vi "WPI_JoystickFindJoystick.vi"(8 "error in (no error)":errorcluster, 9 "Joystick Info":T3, 11 "Match Criteria":T2(array[ring])) -> (0 "error out":errorcluster, 2 "Matching Joysticks":T1[](array[typedef]))   [LabVIEW 2017]
doc: "Search, and return the joystick indices that match the specified criteria.\nName includes is case agnostic, counts match of greater or equal to the critera, and Axis types matches if all criteria are present.\n\nThis software is licensed. Open the labview\\readme\\WPI Robotics Library Open Source License.txt file for more information."
uses:
  <vilib>/Rock Robotics/WPI/Joystick/WPI_Joystick Info.ctl
  <vilib>/Rock Robotics/WPI/Joystick/WPI_JoystickHID Types.ctl
  <vilib>/Rock Robotics/WPI/Joystick/WPI_JoystickXBox Types.ctl
  <vilib>/Rock Robotics/WPI/Joystick/WPI_JoystickAxis Types.ctl
  <vilib>/Rock Robotics/WPI/Joystick/WPI_JoystickDeviceEnum.ctl
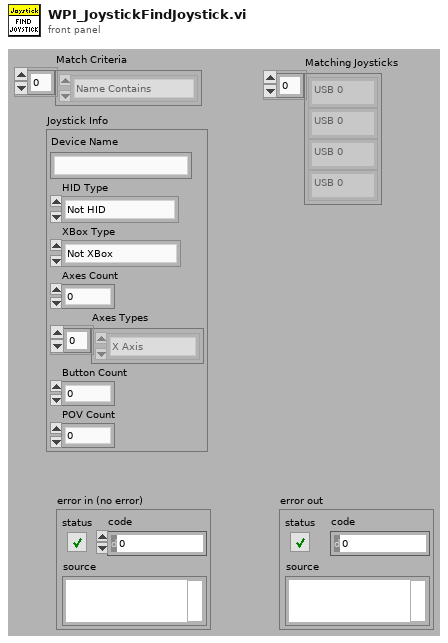
[diagram p1: front panel]
types:
  T1 = typedef "WPI_JoystickDeviceEnum.ctl" = enum16{"USB 0", "USB 1", "USB 2", "USB 3", "USB 4", "USB 5"}
  T2 = enum16{"Name Contains", "Name Equals", "HID Type", "XBox Type", "Axis Count", "Axis Type", "Button Count", "POV Count"}[]
  T3 = typedef "WPI_Joystick Info.ctl" = cluster{"Device Name":string, "HID Type":T4, "XBox Type":T5, "Axes Count":i32, "Axes Types":T6[], "Button Count":i32, "POV Count":i32}
  T4 = typedef "WPI_JoystickHID Types.ctl" = enum16{"Not HID", "HID Joystick", "HID Gamepad", "HID Driving Wheel", "HID Flightstick", "HID First Person"}
  T5 = typedef "WPI_JoystickXBox Types.ctl" = enum16{"Not XBox", "XBox Unknown", "XBox Gamepad", "XBox Wheel", "XBox Arcade Stick", "XBox Flight Stick", "XBox Dance Pad", "XBox Guitar", "XBox Drum Kit", "XBox Arcade Pad"}
  T6 = typedef "WPI_JoystickAxis Types.ctl" = enum16{"X Axis", "Y Axis", "Z Axis", "RxAxis", "RyAxis", "RzAxis", "Slider", "POV", "None", "L X Axis", "L Y Axis", "L Trigger", "R Trigger", "R X Axis", "R Y Axis"}
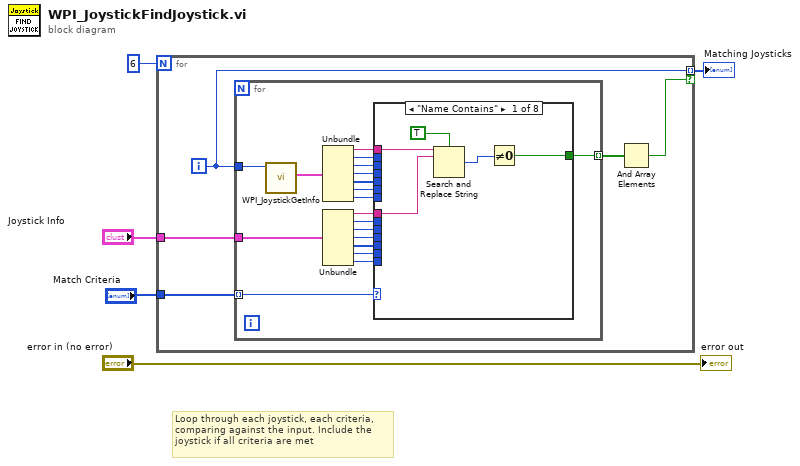
[diagram p0: block diagram]
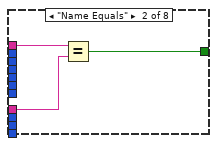
[diagram p2: hidden frame]
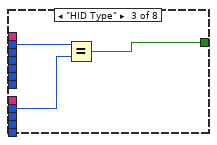
[diagram p3: hidden frame]
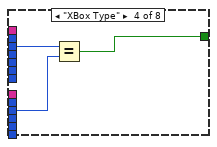
[diagram p4: hidden frame]
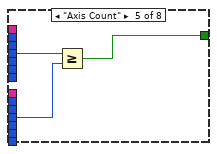
[diagram p5: hidden frame]
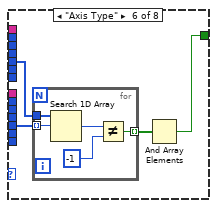
[diagram p6: hidden frame]
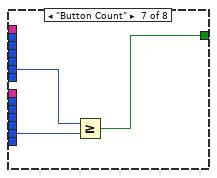
[diagram p7: hidden frame]
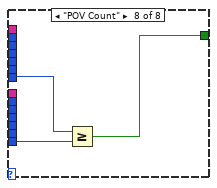
[diagram p8: hidden frame]
diagram:
  # "Loop through each joystick, each criteria,\ncomparing against the input. Include the\njoystick if all criteria are met"
  n1 = for {
    N: 6 -> [_]
    tunnel: "Match Criteria" -> [w10]
    tunnel: "Joystick Info" -> [w9]
    tunnel: [w8] -> w1 mode=indexing if=w6
    i -> [w8]
    n2 = for {
      tunnel: w10 -> [w29] mode=indexing
      tunnel: w9 -> [w28]
      tunnel: [w12] -> w7 mode=indexing
      tunnel: w8 -> [w11]
      n3 = call <vilib>:"WPI_JoystickGetInfo.vi"("JoystickDevice"=w11) -> ("Joystick Info"=w20:T3)  [unwired: 9 in, 1 out]
      n4 = Unbundle(w20) -> ("Device Name"=w19:string, "HID Type"=w18:T4, "XBox Type"=w17:T5, "Axes Count"=w16:i32, "Axes Types"=w15:T6[], "Button Count"=w14:i32, "POV Count"=w13:i32)
      n5 = Unbundle(w28) -> ("Device Name"=w27:string, "HID Type"=w26:T4, "XBox Type"=w25:T5, "Axes Count"=w24:i32, "Axes Types"=w23:T6[], "Button Count"=w22:i32, "POV Count"=w21:i32)
      n6 = case shown="\"Name Contains\"" w29 {
        tunnel: w27 -> [w33 w36 _ _ _ _ _ _]
        tunnel: w26 -> [_ _ w39 _ _ _ _ _]
        tunnel: w25 -> [_ _ _ w42 _ _ _ _]
        tunnel: w24 -> [_ _ _ _ w45 _ _ _]
        tunnel: w23 -> [_ _ _ _ _ w50 _ _]
        tunnel: w22 -> [_ _ _ _ _ _ w56 _]
        tunnel: w21 -> [_ _ _ _ _ _ _ w61]
        tunnel: w19 -> [w34 w37 _ _ _ _ _ _]
        tunnel: w18 -> [_ _ w40 _ _ _ _ _]
        tunnel: w17 -> [_ _ _ w43 _ _ _ _]
        tunnel: w16 -> [_ _ _ _ w46 _ _ _]
        tunnel: w15 -> [_ _ _ _ _ w49 _ _]
        tunnel: w14 -> [_ _ _ _ _ _ w58 _]
        tunnel: w13 -> [_ _ _ _ _ _ _ w60]
        tunnel: [w30 w35 w38 w41 w44 w47 w57 w59] -> w12
        frame "Name Contains" {
          n7 = Search and Replace String(case sensitive?=TRUE, input string=w34, search string=w33) -> (number of replacements=w31:i32)  [unwired: 5 in, 3 out]
          n8 = Not Equal To 0?(x=w31) -> (x != 0?=w30:bool)
        }
        frame "Name Equals" {
          n9 = Equal?(x=w37, y=w36) -> (x = y?=w35:bool)
        }
        frame "HID Type" {
          n10 = Equal?(x=w40, y=w39) -> (x = y?=w38:bool)
        }
        frame "XBox Type" {
          n11 = Equal?(x=w43, y=w42) -> (x = y?=w41:bool)
        }
        frame "Axis Count" {
          n12 = Greater Or Equal?(x=w46, y=w45) -> (x >= y?=w44:bool)
        }
        frame "Axis Type" {
          n13 = for {
            tunnel: w50 -> [w54] mode=indexing
            tunnel: w49 -> [w55]
            tunnel: [w51] -> w48 mode=indexing
            n14 = Search 1D Array(1D array=w55, element=w54) -> (index of element=w53:i32)  [unwired: 1 in]
            n15 = Not Equal?(x=w53, y=-1) -> (x != y?=w51:bool)
          }
          n16 = And Array Elements(Boolean array=w48) -> (logical AND=w47:bool)
        }
        frame "Button Count" {
          n17 = Greater Or Equal?(x=w58, y=w56) -> (x >= y?=w57:bool)
        }
        frame "POV Count" {
          n18 = Greater Or Equal?(x=w60, y=w61) -> (x >= y?=w59:bool)
        }
      }
    }
    n19 = And Array Elements(Boolean array=w7) -> (logical AND=w6:bool)
  }
  "Matching Joysticks" <- w1
  "error out" <- "error in (no error)"
